vi "Monthly Loan Calculator.vi"() -> ()   [LabVIEW 2017]
panel:
  in  "Months":dbl
  in  "Interest Rate":dbl
  in  "Loan Amount":dbl
  out "Monthly Payment":dbl
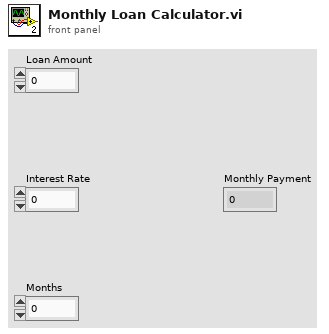
[diagram p1: front panel]
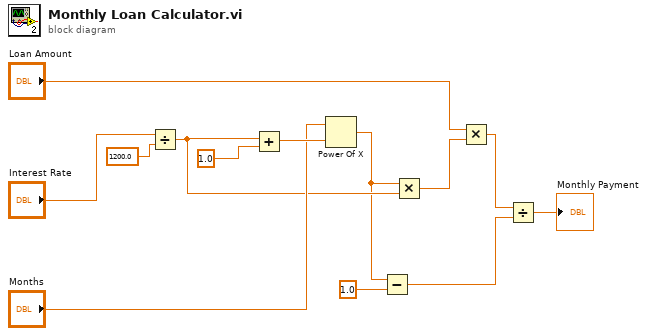
[diagram p0: block diagram]
diagram:
  n1 = Divide(x="Interest Rate", y=1200.0 ("x")) -> (x/y=w7:dbl)
  n2 = Add(x=w7, y=1.0) -> (x+y=w9:dbl)
  n3 = Power Of X(1:w9, 2:"Months") -> (0:w4:dbl)
  n4 = Subtract(x=w4, y=1.0) -> (x-y=w3:dbl)
  n5 = Multiply(x=w4, y=w7) -> (x*y=w6:dbl)
  n6 = Multiply(x="Loan Amount", y=w6) -> (x*y=w2:dbl)
  n7 = Divide(x=w2, y=w3) -> (x/y=→"Monthly Payment":dbl)
